vi "Generate Graph DVR.vi"(8 "Error In":errorcluster, 11 "Graph In":refnum<class "Graph.lvclass">) -> (0 "Error Out":errorcluster, 3 "Graph Out":refnum<class "Graph.lvclass">)   [LabVIEW 2019, in "Graph.lvclass"]
uses:
  Graph.lvclass
  Controls/Data.ctl
  Graph.lvclass/Graph.ctl
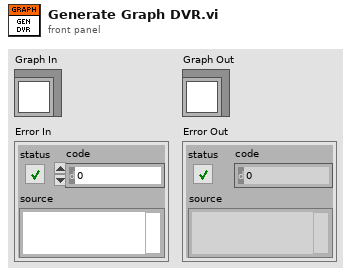
[diagram p1: front panel]
types:
  T1 = typedef "Graph.lvclass/Data.ctl" = cluster{"Height":u32, "Width":u32}
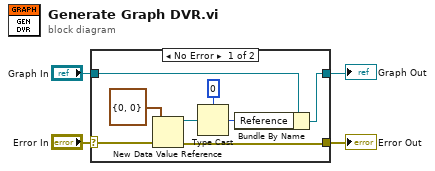
[diagram p0: block diagram]
diagram:
  n1 = case shown="No Error" "Error In" {
    selector: "Error In" -> [w12 w14]
    tunnel: "Graph In" -> [w9 w13]
    tunnel: [w6 w14] -> w3
    tunnel: [w7 w13] -> w1
    frame No Error {
      n2 = New Data Value Reference(data value=T1 {"Height"=0, "Width"=0} ("Data"), error in=w12) -> (data value reference=w10:refnum<data-value>, error out=w6:errorcluster)
      n3 = Type Cast(type=u64 0, x=w10) -> (*(type *) &x=w8:u64)
      n4 = Bundle By Name(cluster=w9, "Reference"=w8) -> (w7:refnum<class "Graph.lvclass">)
    }
    frame Error {
    }
  }
  "Error Out" <- w3
  "Graph Out" <- w1
